vi "Save Image.vi"(8 "error in (no error)":errorcluster, 11 "Save Image in":refnum<class "Save Image.lvclass">) -> (0 "error out":errorcluster, 3 "Save Image out":refnum<class "Save Image.lvclass">)   [LabVIEW 2018, in "Save Image.lvclass"]
uses:
  Save Image.lvclass
  <vilib>/Enthought/Python Integration Toolkit/api/Python Objects.ctl
  Save Image.lvclass/Save Image.ctl
  Channel/Channel.lvclass/Channel.ctl
  Python Toolkit/Python Toolkit.lvclass/Python Toolkit.ctl
  Simulated_CCD_Camera/Simulated_CCD_Camera.lvclass
  Channel/Channel.lvclass
  Python Toolkit/Python Toolkit.lvclass
  <vilib>/Enthought/Python Integration Toolkit/Python Integration Toolkit.lvlib
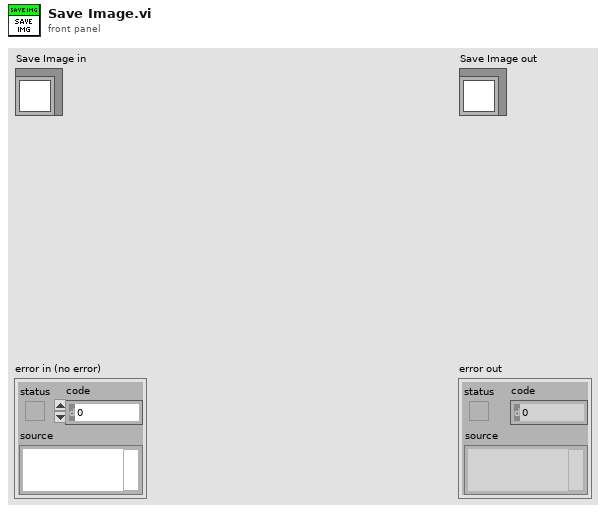
[diagram p1: front panel]
types:
  T1 = typedef "Python Integration Toolkit.lvlib/Python Objects.ctl" = variant
  T2 = cluster{"CUBE_EXPOSURE_TIME":sgl, "CUBES_DONE":u16, "LAST_IMAGE_NAME":string, "DISK_SPACE":u16, "FRAMES_DONE":u16, "CCD_STATUS":string, "CURRENT_TEMPERATURE":i16, "TEMPERATURE_STATUS":string, "FRAME_EXPOSURE_TIME":dbl, "CCD_POWER_STATUS":bool, "SERIAL_NUMBER":u16, "ACQUIRING":bool}
  T3 = cluster{"PREAMP":u16, "READOUT_RATE":u16, "EM_GAIN":u16, "VERTICAL_SHIFT_SPEED":u16, "READ_MODE":u16, "FRAME_TRANSFER":bool, "VERTICAL_CLOCK_VOLTAGE":u16, "ACQUISITION_MODE":u16, "AD_CHANNEL":u16, "EM_MODE":u16, "SHUTTER_TTL":u16, "SHUTTER_OPENING_TIME":u16, "SHUTTER_CLOSING_TIME":u16, "SHUTTER_MODE":u16, "TRIGGER_MODE":u16, "VBIN":u16, "INITIAL_LINE":u16, "INITIAL_COLUMN":u16, "FINAL_LINE":u16, "FINAL_COLUMN":u16, "HBIN":u16}
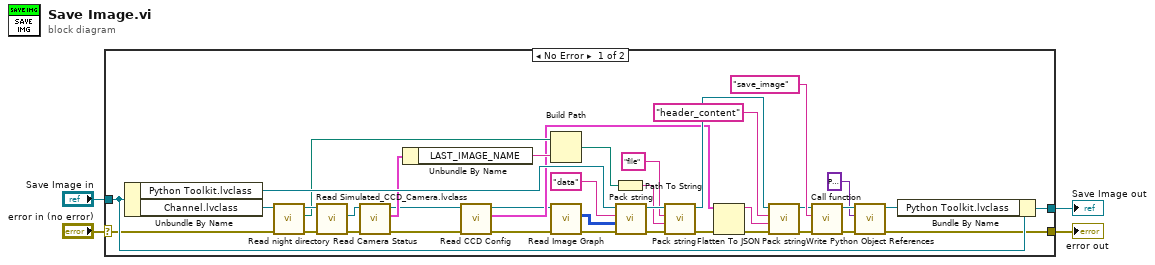
[diagram p0: block diagram]
diagram:
  n1 = case shown="No Error" "error in (no error)" {
    selector: "error in (no error)" -> [w24 w43]
    tunnel: [w32 w43] -> w1
    tunnel: [w41 w44] -> w2
    tunnel: "Save Image in" -> [w42 w44]
    frame No Error {
      n2 = Unbundle By Name(w42) -> ("Python Toolkit.lvclass"=w40:refnum<class "Python Toolkit.lvclass">, "Channel.lvclass"=w25:refnum<class "Channel.lvclass">)
      n3 = call-dynamic "Read night directory.vi"("error in (no error)"=w24, "Channel in"=w25) -> ("error out"=w23:errorcluster, "night directory"=w19:path, "Channel out"=w22:refnum<class "Channel.lvclass">)  [unwired: 7 in]
      n4 = call "Read Simulated_CCD_Camera.lvclass.vi"("error in (no error)"=w23, "Channel in"=w22) -> ("error out"=w26:errorcluster, "Simulated_CCD_Camera.lvclass"=w27:refnum<class "Simulated_CCD_Camera.lvclass">)  [unwired: 7 in, 1 out]
      n5 = call "Read Camera Status.vi"("error in (no error)"=w26, "CCDCamera in"=w27) -> ("error out"=w9:errorcluster, "Camera Status"=w10:T2, "CCDCamera out"=w5:refnum<class "Simulated_CCD_Camera.lvclass">)  [unwired: 7 in]
      n6 = Unbundle By Name(w10) -> ("LAST_IMAGE_NAME"=w20:string)
      n7 = call "Read CCD Config.vi"("error in (no error)"=w9, "CCDCamera in"=w5) -> ("error out"=w8:errorcluster, "CCD Config"=w7:T3, "CCDCamera out"=w6:refnum<class "Simulated_CCD_Camera.lvclass">)  [unwired: 7 in]
      n8 = Build Path(base path=w19, name or relative path=w20) -> (appended path=w21:path)
      n9 = call "Read Image Graph.vi"("error in (no error)"=w8, "CCDCamera in"=w6) -> ("error out"=w29:errorcluster, "Image Graph"=w28:u16[][][])  [unwired: 7 in, 1 out]
      n10 = Path To String(path=w21) -> (string=w18:string)
      n11 = call "Pack string.vi"("error in (no error)"=w29, "Argument"=w28, "Keyword Name"="data", "Python Toolkit in"=w40) -> ("error out"=w38:errorcluster, "Python Toolkit out"=w39:refnum<class "Python Toolkit.lvclass">)  [unwired: 6 in]
      n12 = call "Pack string.vi"("error in (no error)"=w38, "Argument"=w18, "Keyword Name"="file", "Python Toolkit in"=w39) -> ("error out"=w13:errorcluster, "Python Toolkit out"=w17:refnum<class "Python Toolkit.lvclass">)  [unwired: 6 in]
      n13 = Flatten To JSON(anything=w7, error in (no error)=w13) -> (JSON string=w11:string, 11:w12:errorcluster)  [unwired: 1 in]
      n14 = call "Pack string.vi"("error in (no error)"=w12, "Argument"=w11, "Keyword Name"="header_content" ("Function Name"), "Python Toolkit in"=w17) -> ("error out"=w15:errorcluster, "Python Toolkit out"=w16:refnum<class "Python Toolkit.lvclass">)  [unwired: 6 in]
      n15 = call "Call function.vi"("error in (no error)"=w15, "Function Name"="save_image", "Python Toolkit in"=w16) -> ("error out"=w31:errorcluster, "Python Toolkit out"=w34:refnum<class "Python Toolkit.lvclass">)  [unwired: 7 in]
      n16 = call "Write Python Object References.vi"("error in (no error)"=w31, "Python Objects"=T1 variant, "Python Toolkit in"=w34) -> ("error out"=w32:errorcluster, "Python Toolkit out"=w33:refnum<class "Python Toolkit.lvclass">)  [unwired: 7 in]
      n17 = Bundle By Name(cluster=w42, "Python Toolkit.lvclass"=w33) -> (w41:refnum<class "Save Image.lvclass">)
    }
    frame Error {
    }
  }
  "error out" <- w1
  "Save Image out" <- w2
